vi "X-Y-Z-BC-Pro_Api.vi"() -> ()   [LabVIEW 2019]
uses:
  <vilib>/Platform/TimedLoop/XDataNode/wakeup.ctl
  <vilib>/Platform/TimedLoop/XDataNode/XDNodeRunTimeDep.lvlib
  <vilib>/Platform/TimedLoop/XDataNode/nitl_modes.ctl
  <vilib>/Platform/TimedLoop/XDataNode/timing_clust.ctl
  <vilib>/platform/TimedLoop/XDataNode/XDataNode.xnode
panel:
  in  "X-Y-Z移動 2":dbl[][](array[numeric])=[[0.0, 0.0, 0.0, 0.0], [0.0, 0.0, 0.0, 0.0], [0.0, 0.0, 0.0, 0.0]]
  in  "加速度":dbl=800.0
  in  "最高速":dbl=1150.0
  in  "X-Y-Z移動":dbl[](array[numeric])=[0.0, 0.0, 0.0]
  out "Error Out":errorcluster
  in  "Error In":errorcluster
  out "三角形?":bool
  in  "Stop":bool
  out "Waveform Chart":dbl(graph)
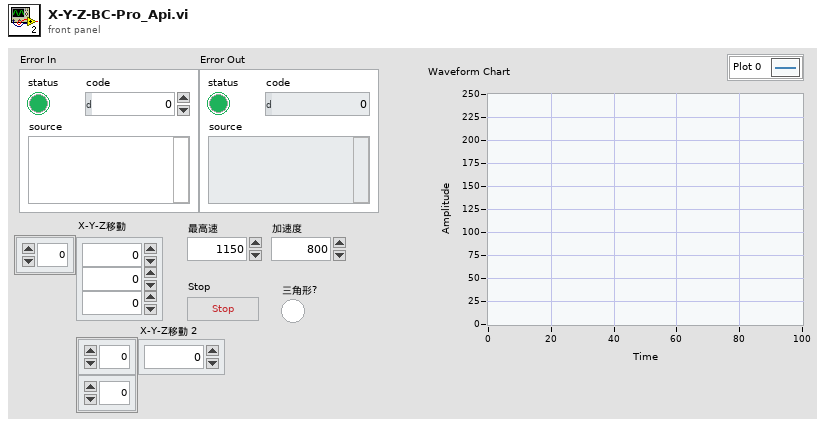
[diagram p1: front panel]
types:
  T1 = typedef "XDNodeRunTimeDep.lvlib/timing_clust.ctl" = cluster{"Expected End [f-1]":u64, "Actual End [f-1]":u64, "Finished Late? [f-1]":bool, "Expected End [i-1]":u64, "Actual End [i-1]":u64, "Finished Late? [i-1]":bool, "Expected Start [i]":u64, "Actual Start [i]":u64, "Expected Start [f]":u64, "Actual Start [f]":u64, "Source Name":string, "Structure Name":string, "Period":i64, "Deadline":i64, "Offset":i64, "Start":i64, "Priority":i32, "Timeout":i32, "Mode":T2, "Wakeup Reason":T3, "Error":errorcluster, "Source Type":string, "Secondary Source Type":string, "Global End Time":u64, "Global Start Time":u64, "Frame Duration":u64, "Iteration Duration":u64, "Assigned CPU":i32, "I/O Scan Engine Mode":u32}
  T2 = typedef "XDNodeRunTimeDep.lvlib/nitl_modes.ctl" = enum32{"No Change", "Process missed periods, maintain original phase", "Discard missed periods, maintain original phase", "Process missed periods, ignore original phase", "Discard missed periods, ignore original phase"}
  T3 = typedef "XDNodeRunTimeDep.lvlib/wakeup.ctl" = enum32{"Normal", "Aborted", "Asynchronous wakeup", "Timing source error", "Timed loop error", "Timeout"}
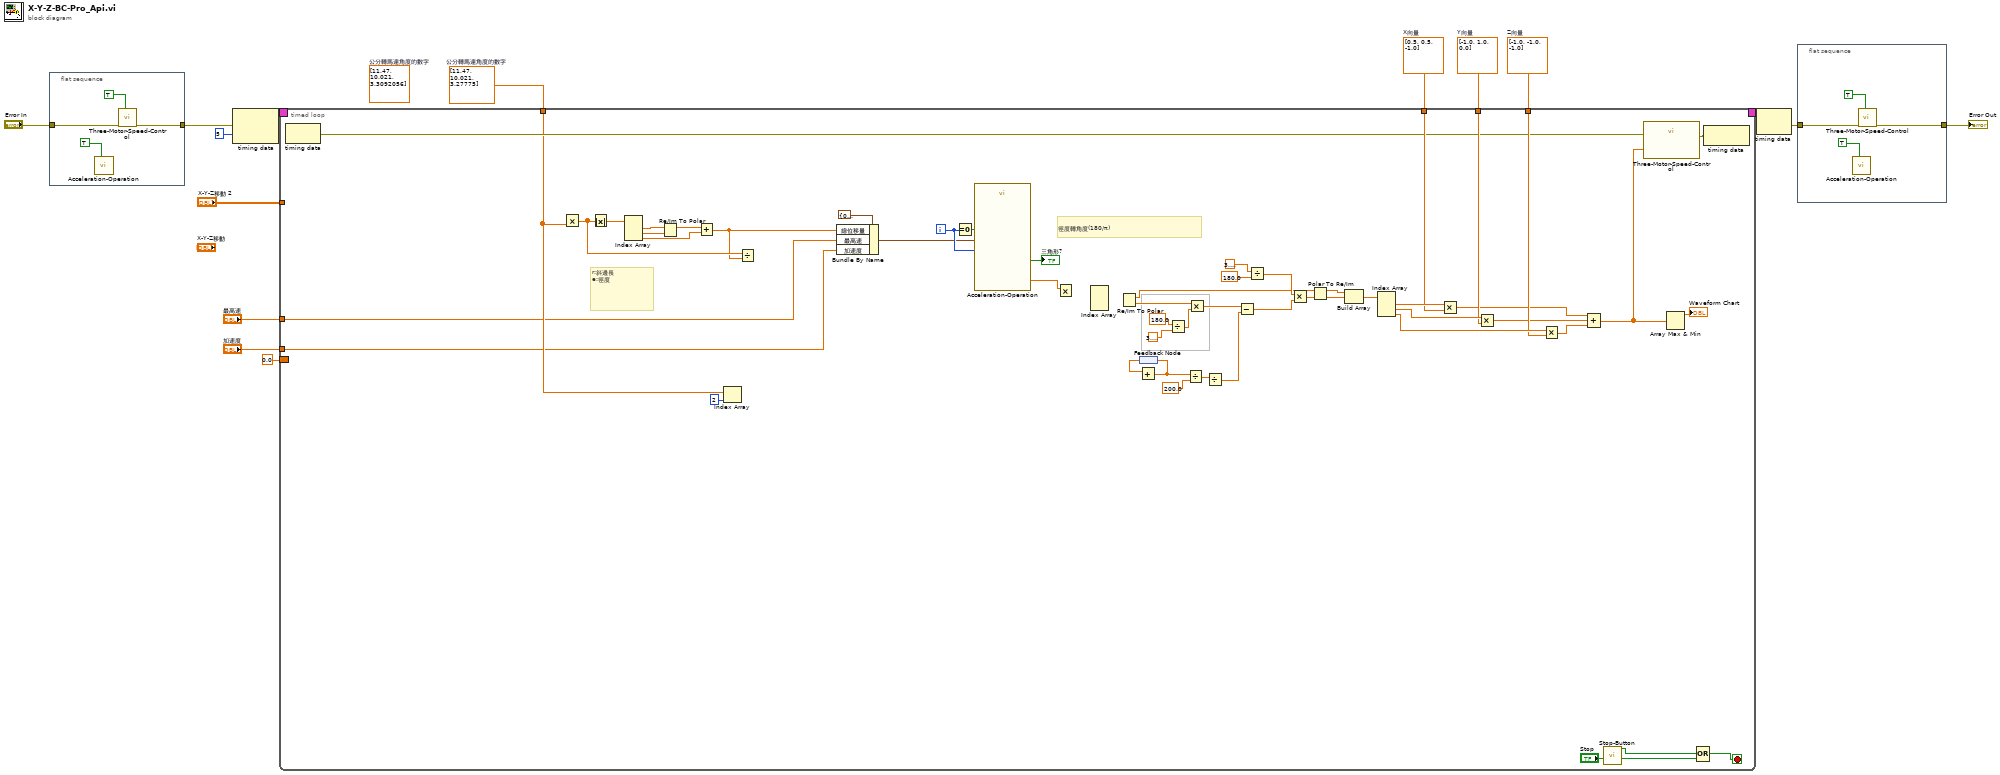
[diagram p0: block diagram]
diagram:
  w3 = dbl[] [11.47, 10.021, 3.27775]  # 公分轉馬達角度的數字
  (unwired) dbl[] [11.47, 10.021, 3.3092056]  # 公分轉馬達角度的數字
  w8 = dbl[] [-1.0, -1.0, -1.0]  # Z向量
  w9 = dbl[] [-1.0, 1.0, 0.0]  # Y向量
  w10 = dbl[] [0.5, 0.5, -1.0]  # X向量
  n1 = flat-sequence {
    tunnel: "Error In" -> [w18]
    tunnel: [w17] -> w12
    frame #0 {
      n2 = call "Acceleration-Operation.vi"("Reset"=TRUE) -> ()  [unwired: 8 in, 3 out]
      n3 = call "Three-Motor-Speed-Control.vi"("Reset"=TRUE, "Error In"=w18) -> ("Error Out"=w17:errorcluster)  [unwired: 9 in]
    }
  }
  n4 = node-c288(w12, i64 5 ("Period")) -> (w15:T1)
  n5 = timed-loop "Timed Loop" {
    timing: w15 -> [_]
    timing-out: [_] -> w14
    border: 0.0 -> [_]
    tunnel: w10 -> [w47]
    tunnel: w9 -> [w45]
    tunnel: w8 -> [w43]
    tunnel: "X-Y-Z移動 2" -> [_]
    tunnel: w3 -> [w22]
    tunnel: "最高速" -> [w21]
    tunnel: "加速度" -> [w20]
    i -> [w69]
    stop <- w67 stop-if-true
    # "r:斜邊長\ne:徑度"
    # "徑度轉角度(180/π)"
    n6 = node-c288() -> (w38:errorcluster)  [unwired: 1 in]
    n7 = Multiply(y=w22) -> (x*y=w32:dbl[])  [unwired: 1 in]
    n8 = Absolute Value(x=w32) -> (abs(x)=w26:dbl[])
    n9 = Index Array(array=w26) -> (element #1=w29:dbl, element #2=w25:dbl, element #3=w28:dbl)  [unwired: 3 in]
    n10 = Re/Im To Polar(2:w25, 3:w29) -> (1:w27:dbl)  [unwired: 1 out]
    n11 = Add(x=w27, y=w28) -> (x+y=w31:dbl)
    n12 = Index Array(array=w22, index=2) -> ()  [unwired: 1 out]
    n13 = Divide(x=w32, y=w31) -> ()  [unwired: 1 out]
    n14 = Bundle By Name(cluster=cluster{"總位移量":dbl, "最高速":dbl, "加速度":dbl} {"總位移量"=0.0, "最高速"=0.0, "加速度"=0.0} ("計算設置"), "總位移量"=w31, "最高速"=w21, "加速度"=w20) -> (w24:cluster{"總位移量":dbl, "最高速":dbl, "加速度":dbl})
    n15 = Equal To 0?(x=w69) -> (x = 0?=w70:bool)
    n16 = call "Acceleration-Operation.vi"("Reset"=w70, "迴圈( I )"=w69, "計算設置"=w24) -> ("速度"=w71:dbl, "三角形?"=→"三角形?":bool)  [unwired: 6 in, 1 out]
    n17 = Multiply(x=w71) -> ()  [unwired: 1 in, 1 out]
    n18 = Index Array() -> ()  [unwired: 4 in, 3 out]
    n19 = Re/Im To Polar() -> (0:w65:dbl, 1:w52:dbl)  [unwired: 2 in]
    n20 = feedback #1() -> (w61:dbl)
    n21 = Add(x=w61) -> (x+y=w60:dbl)  [unwired: 1 in]
    n22 = feedback-in #1(w60) -> ()
    n23 = Divide(x=180.0, y=3.141592653589793) -> (x/y=w62:dbl)
    n24 = Divide(x=w60, y=200.0) -> (x/y=w37:dbl)
    n25 = Multiply(x=w65, y=w62) -> (x*y=w58:dbl)
    n26 = Divide(x=w37) -> (x/y=w36:dbl)  [unwired: 1 in]
    n27 = Subtract(x=w58, y=w36) -> (x-y=w54:dbl)
    n28 = Divide(x=3.141592653589793, y=180.0 ("x")) -> (x/y=w55:dbl)
    n29 = Multiply(x=w55, y=w54) -> (x*y=w53:dbl)
    n30 = Polar To Re/Im(2:w53, 3:w52) -> (0:w50:dbl, 1:w51:dbl)
    n31 = Build Array(w51, w50) -> (w49:dbl[])  [unwired: 1 in]
    n32 = Index Array(array=w49) -> (element #1=w48:dbl, element #2=w46:dbl, element #3=w44:dbl)  [unwired: 3 in]
    n33 = Multiply(x=w48, y=w47) -> (x*y=w42:dbl[])
    n34 = Multiply(x=w46, y=w45) -> (x*y=w41:dbl[])
    n35 = Multiply(x=w44, y=w43) -> (x*y=w40:dbl[])
    n36 = Compound Arithmetic op=ADD(w42, w41, w40) -> (w23:dbl[])
    n37 = call "Stop-Button.vi"() -> ("顯示按下?"=w34:bool)  [unwired: 10 in, 1 out]
    n38 = call "Three-Motor-Speed-Control.vi"("Error In"=w38, "速度(秒/度)"=w23) -> ("Error Out"=w39:errorcluster)  [unwired: 9 in]
    n39 = Array Max & Min(array=w23) -> (max value=→"Waveform Chart":dbl)  [unwired: 3 out]
    n40 = Compound Arithmetic op=OR(w34, "Stop") -> (w67:bool)  [unwired: 1 in]
    n41 = node-c288(w39) -> ()  [unwired: 1 out]
  }
  n42 = node-c288(w14) -> (w7:errorcluster)
  n43 = flat-sequence {
    tunnel: [w80] -> w6
    tunnel: w7 -> [w77]
    frame #0 {
      n44 = call "Acceleration-Operation.vi"("Reset"=TRUE) -> ()  [unwired: 8 in, 3 out]
      n45 = call "Three-Motor-Speed-Control.vi"("Reset"=TRUE, "Error In"=w77) -> ("Error Out"=w80:errorcluster)  [unwired: 9 in]
    }
  }
  "Error Out" <- w6
